vi "CS-4 Get Ranges.vi"(4 "error in":errorcluster, 7 "VISA session":refnum<visa-resource-name>) -> (0 "error out":errorcluster, 1 "range 1":dbl format="%.2f", 2 "range 0":dbl format="%.2f", 3 "dup VISA session":refnum<visa-resource-name>)   [LabVIEW 2016]
doc: "CS-4 Get Ranges.vi will return the sweep ranges."
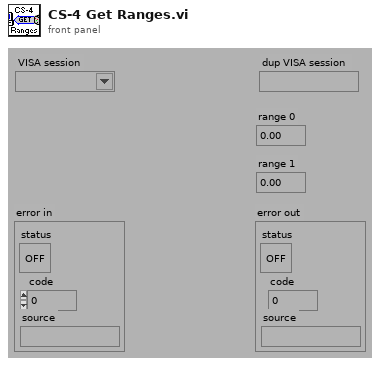
[diagram p1: front panel]
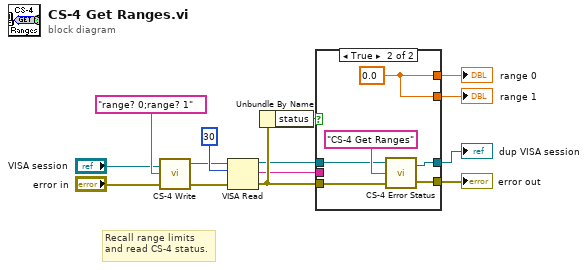
[diagram p0: block diagram]
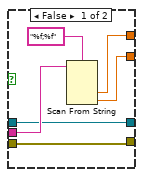
[diagram p2: hidden frame]
diagram:
  # "Recall range limits\nand read CS-4 status."
  n1 = call "CS-4 Write.vi"("error in (no error)"="error in", "write buffer (\"\")"="range? 0;range? 1", "VISA session"="VISA session") -> ("error out"=w5:errorcluster, "dup VISA session"=w4:refnum<visa-resource-name>)  [unwired: 1 out]
  n2 = VISA Read(VISA resource name=w4, byte count=u32 30 ("byte count (0)"), error in (no error)=w5) -> (VISA resource name out=w10:refnum<visa-resource-name>, read buffer=w9:string, error out=w11:errorcluster)  [unwired: 1 out]
  n3 = Unbundle By Name(w11) -> ("status"=w8:bool)
  n4 = case shown="True" w8 {
    tunnel: w9 -> [w20 _]
    tunnel: w10 -> [w15 w25]
    tunnel: w11 -> [w18 w24]
    tunnel: [w18 w23] -> w12
    tunnel: [w17 w22] -> w13
    tunnel: [w16 w22] -> w14
    tunnel: [w15 w21] -> w1
    frame False {
      n5 = Scan From String(format string="%f;%f", input string=w20) -> (output 1=w17:dbl, output 2=w16:dbl)  [unwired: 4 in, 3 out]
    }
    frame True {
      w22 = 0.0
      n6 = call "CS-4 Error Status.vi"("error in (no error)"=w24, "VI name"="CS-4 Get Ranges", "VISA session"=w25) -> ("error out"=w23:errorcluster, "dup VISA session"=w21:refnum<visa-resource-name>)
    }
  }
  "range 1" <- w14
  "range 0" <- w13
  "error out" <- w12
  "dup VISA session" <- w1
